vi "Bode magnitude plot.vi"() -> ()   [LabVIEW 2015]
uses:
  <vilib>/Analysis/NI_AALPro.lvlib
panel:
  out "XY Graph":cluster{dbl[], dbl[]}(graph)
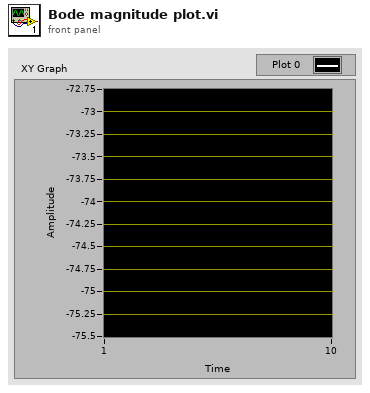
[diagram p1: front panel]
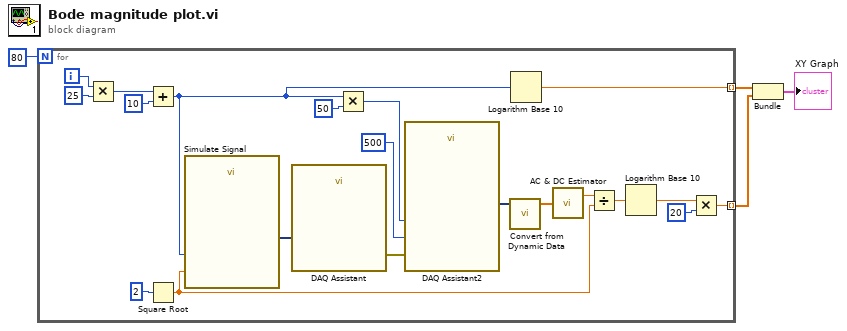
[diagram p0: block diagram]
diagram:
  n1 = for {
    N: 80 -> [_]
    tunnel: [w6] -> w3 mode=indexing
    tunnel: [w5] -> w2 mode=indexing
    i -> [w10]
    n2 = Multiply(x=w10, y=25) -> (x*y=w15:i32)
    n3 = Add(x=w15, y=10) -> (x+y=w9:i32)
    n4 = Square Root(x=2) -> (sqrt(x)=w12:dbl)
    n5 = call "Simulate Signal"("Frequency"=w9, "Amplitude"=w12) -> ("Sine"=w24:dynamicdata)  [unwired: 12 in, 1 out]
    n6 = call "DAQ Assistant"("data"=w24) -> ("error out"=w23:errorcluster)  [unwired: 16 in, 2 out]
    n7 = Multiply(x=w9, y=50) -> (x*y=w19:i32)
    n8 = call "DAQ Assistant2"("rate"=w19, "number of samples"=500, "error in"=w23) -> ("data"=w18:dynamicdata)  [unwired: 14 in, 2 out]
    n9 = call "Convert from Dynamic Data"("Dynamic Data Type"=w18) -> ("Array"=w17:dbl[])  [unwired: 3 in]
    n10 = Logarithm Base 10(1:w9) -> (0:w6:dbl)
    n11 = call <vilib>:"AC & DC Estimator.vi"("Signal (V)"=w17) -> ("AC estimate (Vrms)"=w13:dbl)  [unwired: 1 out]
    n12 = Divide(x=w13, y=w12) -> (x/y=w8:dbl)
    n13 = Logarithm Base 10(1:w8) -> (0:w7:dbl)
    n14 = Multiply(x=w7, y=20) -> (x*y=w5:dbl)
  }
  n15 = Bundle(w3, w2) -> (→"XY Graph":cluster{dbl[], dbl[]})  [unwired: 1 in]
